vi "FM_RTL-SDR_RX_MATLAB_Script.vi"() -> (3 "Calculation Time (s)":dbl)   [LabVIEW 2013]
doc: "Demonstrates how to use the MATLAB script node. The m-file script is used to calculate the data and the resulting fractal is displayed on the front panel. The MathWorks, Inc. MATLAB (R) Application Software version 5.0 or later must be installed and properly licensed in order to run this VI."
uses:
  <vilib>/Waveform/WDTFileIO.llb/Read Waveform from File.vi
panel:
  out "Baseband":dbl[](array[numeric])
  in  "file path":path=path "D:/File/Recoder_Data_IQIQ"
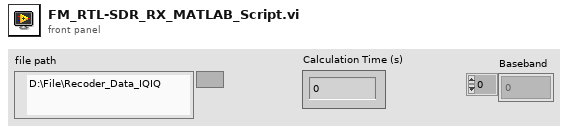
[diagram p1: front panel]
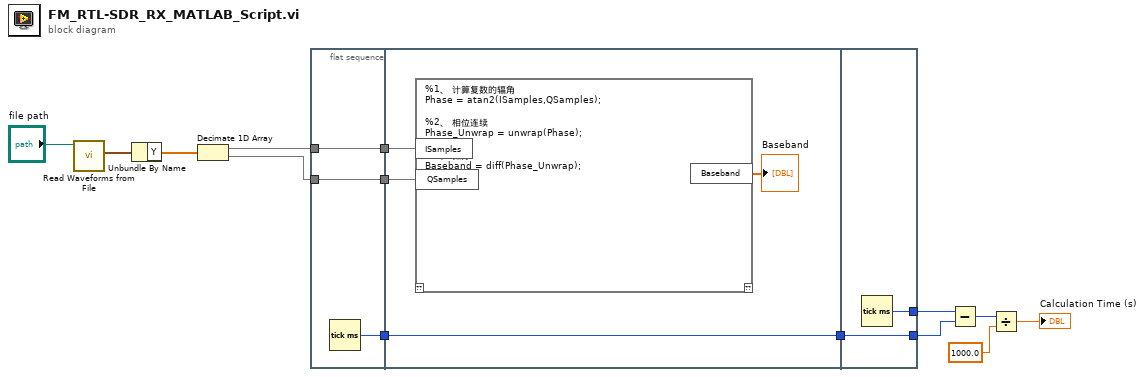
[diagram p0: block diagram]
diagram:
  n1 = call-poly <vilib>:"Read Waveforms from File.vi"("file path (dialog if empty)"="file path") -> ("first waveform in record"=w7:waveform(dbl))  [unwired: 5 in, 3 out]
  n2 = Unbundle By Name(w7) -> ("Y"=w5:dbl[])
  n3 = Decimate 1D Array(w5) -> (w3:dbl[], w2:dbl[])
  n4 = flat-sequence {
    tunnel: [w17] -> w8
    tunnel: [w16] -> w4
    tunnel: w3 -> [w16]
    tunnel: w2 -> [w15]
    tunnel: [w15] -> w1
    tunnel: [w21] -> w14
    tunnel: w8 -> [w21]
    tunnel: w4 -> [w20]
    tunnel: w1 -> [w19]
    tunnel: w14 -> [w22]
    tunnel: [w23] -> w11
    tunnel: [w22] -> w10
    frame #0 {
      n5 = Tick Count (ms)() -> (millisecond timer value=w17:u32)
    }
    frame #1 {
      n6 = script code="%1、 计算复数的辐角\nPhase = atan2(ISamples,QSamples);\n\n%2、 相位连续\nPhase_Unwrap = unwrap(Phase);\n\n%3、 微分\nBaseband = diff(Phase_Unwrap);"("ISamples"=w20, "QSamples"=w19) -> ("Baseband"=→"Baseband":dbl[])  [unwired: 1 in, 1 out]
    }
    frame #2 {
      n7 = Tick Count (ms)() -> (millisecond timer value=w23:u32)
    }
  }
  n8 = Subtract(x=w11, y=w10) -> (x-y=w12:u32)
  n9 = Divide(x=w12, y=1000.0) -> (x/y=→"Calculation Time (s)":dbl)
